vi "GetCarType.vi"(8 "Error In":errorcluster, 11 "reference in":refnum<class "Hatchback.lvclass">) -> (0 "Error Out":errorcluster, 2 "Car Type":string, 3 "reference out":refnum<class "Hatchback.lvclass">)   [LabVIEW 2024, in "Hatchback.lvclass"]
uses:
  Hatchback.lvclass
  Hatchback.lvclass/Hatchback.ctl
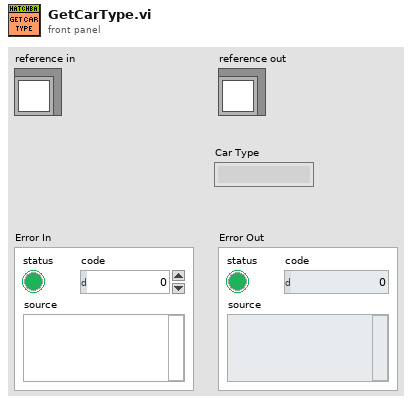
[diagram p1: front panel]
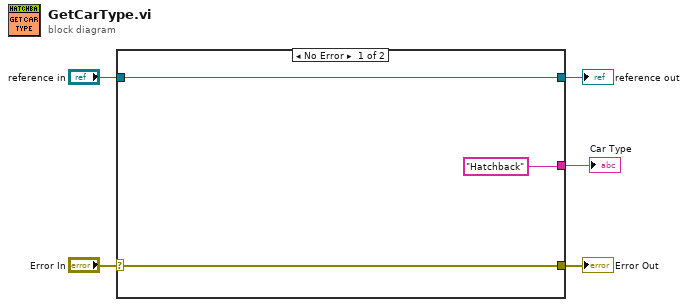
[diagram p0: block diagram]
diagram:
  n1 = case shown="No Error" "Error In" {
    selector: "Error In" -> [w7 w10]
    tunnel: [w7 w10] -> w4
    tunnel: [w8 w9] -> w2
    tunnel: "reference in" -> [w8 w9]
    tunnel: ["Hatchback" _] -> w1
    frame No Error {
    }
    frame Error {
    }
  }
  "Error Out" <- w4
  "reference out" <- w2
  "Car Type" <- w1
